vi "DidStop.vi"(6 "Wait for Module to stop?":bool, 7 "Exit via Stop Module Req?":bool, 8 "error in (no error)":errorcluster, 11 "ModuleAdmin":refnum<class "ModuleAdmin.lvclass">) -> (0 "error out":errorcluster)   [LabVIEW 2017, in "OutputToFileModule.lvlib"]
uses:
  OutputToFileModule.lvlib
  <userlib>/NIST/ModuleAdminLib/ModuleAdmin/ModuleAdmin.lvclass
  PublicAPI/Arguments/Requests/clStopArgument.ctl
  Private/clEventType.ctl
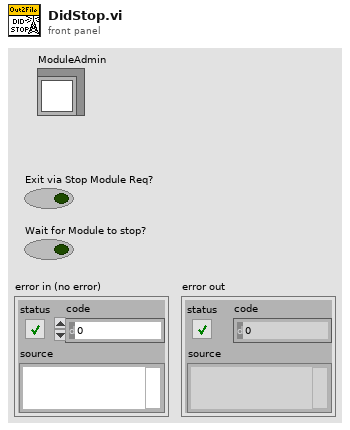
[diagram p1: front panel]
types:
  T1 = typedef "OutputToFileModule.lvlib/clEventType.ctl" = cluster{"ModuleID":i32, "Data":variant}
  T2 = typedef "OutputToFileModule.lvlib/clStopArgument.ctl" = cluster{"Exit via Stop Module Req?":bool, "Wait for Module to stop?":bool, "ModuleAdmin":refnum<class "ModuleAdmin.lvclass">}
  T3 = typedef "OutputToFileModule.lvlib/clBroadcastEvents.ctl" = cluster{"DidInit":refnum<user-event>, "StatusUpdate":refnum<user-event>, "ErrorReport":refnum<user-event>, "DidStop":refnum<user-event>, "PathToPlugin":refnum<user-event>, "PmuConfig":refnum<user-event>, "OutputPath":refnum<user-event>}
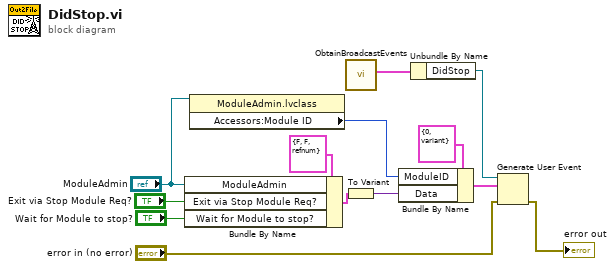
[diagram p0: block diagram]
diagram:
  n1 = Bundle By Name(cluster=T2 {"Exit via Stop Module Req?"=FALSE, "Wait for Module to stop?"=FALSE, "ModuleAdmin"=refnum} ("Stop Argument"), "ModuleAdmin"="ModuleAdmin", "Exit via Stop Module Req?"="Exit via Stop Module Req?", "Wait for Module to stop?"="Wait for Module to stop?") -> (w11:T2)
  n2 = property class="ModuleAdmin.lvclass"(reference="ModuleAdmin") -> ("Accessors:Module ID"=w1:i32)  [unwired: 1 in, 2 out]
  n3 = call "ObtainBroadcastEvents.vi"() -> ("clBroadcastEvents"=w12:T3)  [unwired: 10 in, 1 out]
  n4 = To Variant(anything=w11) -> (Variant=w8:variant)
  n5 = Bundle By Name(cluster=T1 {"ModuleID"=0, "Data"=variant} ("clBroadcast"), "ModuleID"=w1, "Data"=w8) -> (w7:T1)
  n6 = Unbundle By Name(w12) -> ("DidStop"=w10:refnum<user-event>)
  n7 = Generate User Event(user event=w10, event data cluster=w7, error in="error in (no error)") -> (error out=→"error out":errorcluster)  [unwired: 1 in, 1 out]
